vi "process_DAQ.vi"(8 "error in (no error)":errorcluster) -> (0 "error out":errorcluster)   [LabVIEW 2010]
uses:
  typedefs/control_daq_enum.ctl
  typedefs/data_array.ctl
  typedefs/acquisition_parameters_cluster.ctl
  typedefs/stimulation_parameters.ctl
  C:/Program Files (x86)/National Instruments/LabVIEW 2010/vi.lib/ULx/ULx_LV.dll
  Program Files (x86)/National Instruments/LabVIEW 2010/vi.lib/ULx/ULx_LV.dll
  <vilib>/ULx/Read.llb/ULx Read (Analog 2D DBL NChan NSamp).vi
panel:
  out "Package start time":timestamp format="%<%.3X>T"
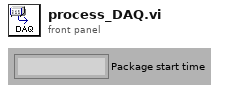
[diagram p1: front panel]
types:
  T1 = typedef "control_daq_enum.ctl" = enum16{"Init", "GetCont", "GetNoSamples", "Stop", "Quit"}
  T2 = cluster{"Control DAQ Enum":T1, "variant":variant}
  T3 = typedef "data_array.ctl" = waveform(dbl)[]
  T4 = typedef "acquisition_parameters_cluster.ctl" = cluster{"Physical channels":refnum<k21>, "Shutter line":refnum<k21>, "Clock source":i32, "Triggered?":bool, "Sample rate":dbl, "Pixels to integrate":i32, "Effective data rate":dbl, "Read chunk size":i32, "Samples to read":i32, "Run mode":enum32{"Continuously", "Fixed sample number"}}
  T5 = typedef "stimulation_parameters.ctl" = cluster{"Physical channel":tag, "Write chunk size":i32, "Sample rate":dbl, "Stim onset":dbl, "Stim frequency":dbl, "ON time":dbl, "OFF time":dbl, "Repetitions":dbl}
  T6 = cluster{"Acquisition parameters":T4, "Stimulation parameters":T5}
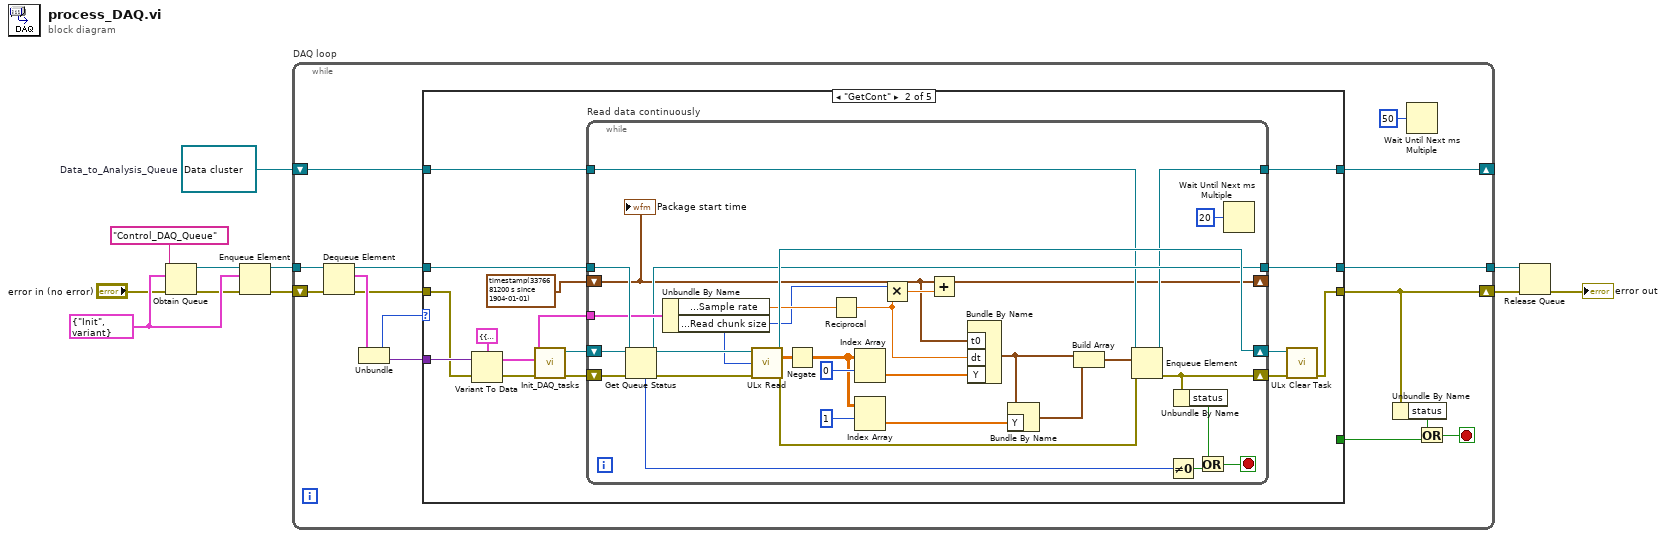
[diagram p0: block diagram]
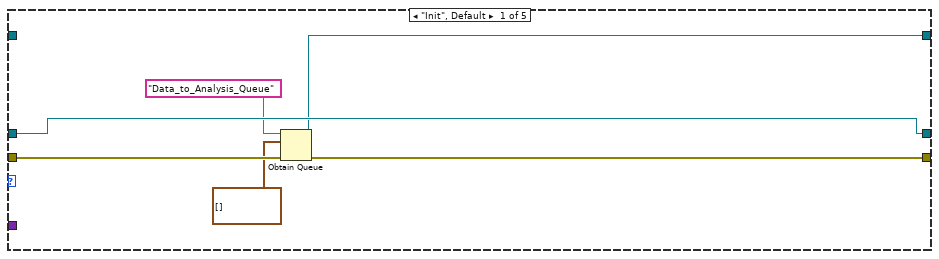
[diagram p2: hidden frame]
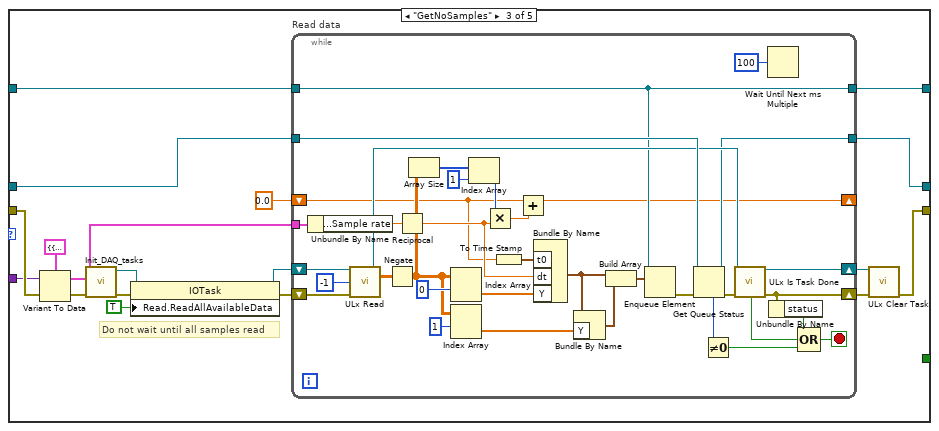
[diagram p3: hidden frame]
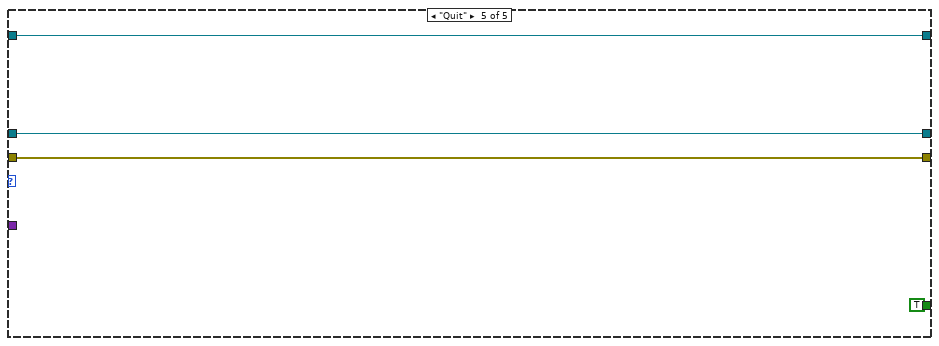
[diagram p5: hidden frame]
diagram:
  w1 = refnum<queue> refnum  # Data_to_Analysis_Queue
  w11 = T2 {"Control DAQ Enum"=enum."Init", "variant"=variant} ("ControlDAQ state cluster")
  n1 = Obtain Queue(name (unnamed)="Control_DAQ_Queue", element data type=w11, error in (no error)="error in (no error)") -> (queue out=w7:refnum<queue>, error out=w9:errorcluster)  [unwired: 2 in, 1 out]
  n2 = Enqueue Element(queue=w7, element=w11, error in (no error)=w9) -> (queue out=w8:refnum<queue>, error out=w10:errorcluster)  [unwired: 1 in, 1 out]
  n3 = while "DAQ loop" {
    shift-right: [w19] -> w6
    shift-left: w10 -> [w25]
    tunnel: w8 -> [w26]
    tunnel: [w15] -> w5
    shift-right: [w13] -> _
    shift-left: w1 -> [w14]
    stop <- w17 stop-if-true
    n4 = Dequeue Element(queue=w26, error in (no error)=w25) -> (queue out=w24:refnum<queue>, element=w23:T2, error out=w21:errorcluster)  [unwired: 1 in, 1 out]
    n5 = Unbundle(w23) -> ("Control DAQ Enum"=w16:T1, "variant"=w22:variant)
    n6 = case shown="\"GetCont\"" w16 {
      tunnel: w24 -> [w32 w47 w91 w134 w137]
      tunnel: w22 -> [_ w46 w92 _ _]
      tunnel: w21 -> [w31 w45 w93 w135 w138]
      tunnel: [w29 w34 w90 w135 w138] -> w19
      tunnel: [_ _ _ _ TRUE] -> w20
      tunnel: [w32 w38 w82 w134 w137] -> w15
      tunnel: w14 -> [_ w37 w81 w133 w136]
      tunnel: [w27 w36 w80 w133 w136] -> w13
      frame "Init", Default {
        n7 = Obtain Queue(name (unnamed)="Data_to_Analysis_Queue", element data type=T3 [] ("Data cluster"), error in (no error)=w31) -> (queue out=w27:refnum<queue>, error out=w29:errorcluster)  [unwired: 2 in, 1 out]
      }
      frame "GetCont" {
        n8 = Variant To Data(error in=w45, Variant=w46, type=T6 {"Acquisition parameters"={"Physical channels"="", "Shutter line"="", "Clock source"=0, "Triggered?"=FALSE, "Sample rate"=0.0, "Pixels to integrate"=0, "Effective data rate"=0.0, "Read chunk size"=0, "Samples to read"=0, "Run mode"=enum."Continuously"}, "Stimulation parameters"={"Physical channel"="", "Write chunk size"=0, "Sample rate"=0.0, "Stim onset"=0.0, "Stim frequency"=0.0, "ON time"=0.0, "OFF time"=0.0, "Repetitions"=0.0}} ("output cluster")) -> (error out=w44:errorcluster, data=w41:T6)
        n9 = call "Init_DAQ_tasks.vi"("error in"=w44, "Parameter cluster"=w41) -> ("error out"=w43:errorcluster, "Acq task out"=w42:refnum<k24>)  [unwired: 6 in]
        n10 = while "Read data continuously" {
          shift-right: [w65] -> w39
          shift-left: w43 -> [w69]
          tunnel: w41 -> [w72]
          shift-right: [w73] -> w40
          shift-left: w42 -> [w76]
          shift-right: [w51] -> _
          shift-left: timestamp(3376681200 s since 1904-01-01) ("time stamp") -> [w48]
          tunnel: w37 -> [w70]
          tunnel: [w67] -> w36
          tunnel: w47 -> [w78]
          tunnel: [w71] -> w38
          stop <- w74 stop-if-true
          n11 = Get Queue Status(queue=w78, error in (no error)=w69) -> (queue out=w71:refnum<queue>, error out=w66:errorcluster, # elements in queue=w77:i32)  [unwired: 1 in, 5 out]
          n12 = Unbundle By Name(w72) -> ("Acquisition parameters.Sample rate"=w57:dbl, "Acquisition parameters.Read chunk size"=w49:i32)
          n13 = call-poly <vilib>:"ULx Read.vi"("task in"=w76, "number of samples per channel"=w49, "error in"=w66) -> ("task out"=w73:refnum<k24>, "data"=w68:dbl[][], "error out"=w54:errorcluster)  [unwired: 10 in]
          n14 = Negate(x=w68) -> (-x=w60:dbl[][])
          n15 = Reciprocal(x=w57) -> (1/x=w50:dbl)
          n16 = Index Array(array=w60, index (row)=0) -> (element=w56:dbl[])  [unwired: 1 in]
          n17 = Index Array(array=w60, index (row)=1) -> (element=w59:dbl[])  [unwired: 1 in]
          n18 = Multiply(x=w49, y=w50) -> (x*y=w53:dbl)
          n19 = Add(x=w48, y=w53) -> (x+y=w51:timestamp)
          n20 = Bundle By Name("t0"=w48, "dt"=w50, "Y"=w56) -> (w55:waveform(dbl))  [unwired: 1 in]
          n21 = Bundle By Name(cluster=w55, "Y"=w59) -> (w58:waveform(dbl))
          n22 = Build Array(w55, w58) -> (w52:waveform(dbl)[])
          n23 = Enqueue Element(queue=w70, element=w52, error in (no error)=w54) -> (queue out=w67:refnum<queue>, error out=w65:errorcluster)  [unwired: 1 in, 1 out]
          n24 = Not Equal To 0?(x=w77) -> (x != 0?=w75:bool)
          n25 = Unbundle By Name(w65) -> ("status"=w64:bool)
          n26 = Or(x=w64, y=w75) -> (x .or. y?=w74:bool)
          n27 = Wait Until Next ms Multiple(millisecond multiple=u32 20) -> ()  [unwired: 1 out]
          "Package start time" <- w48
        }
        n28 = call <vilib>:"ULx Clear Task.vi"("task in"=w40, "error in"=w39) -> ("error out"=w34:errorcluster)  [unwired: 13 in]
      }
      frame "GetNoSamples" {
        # "Do not wait until all samples read"
        n29 = Variant To Data(error in=w93, Variant=w92, type=T6 {"Acquisition parameters"={"Physical channels"="", "Shutter line"="", "Clock source"=0, "Triggered?"=FALSE, "Sample rate"=0.0, "Pixels to integrate"=0, "Effective data rate"=0.0, "Read chunk size"=0, "Samples to read"=0, "Run mode"=enum."Continuously"}, "Stimulation parameters"={"Physical channel"="", "Write chunk size"=0, "Sample rate"=0.0, "Stim onset"=0.0, "Stim frequency"=0.0, "ON time"=0.0, "OFF time"=0.0, "Repetitions"=0.0}} ("output cluster")) -> (error out=w96:errorcluster, data=w84:T6)
        n30 = call "Init_DAQ_tasks.vi"("error in"=w96, "Parameter cluster"=w84) -> ("error out"=w87:errorcluster, "Acq task out"=w89:refnum<k24>)  [unwired: 6 in]
        n31 = property class="IOTask"(reference=w89, error in=w87, "Read.ReadAllAvailableData"=TRUE) -> (reference out=w88:refnum<k24>, error out=w86:errorcluster)
        n32 = while "Read data" {
          shift-right: [w124] -> w94
          shift-left: w86 -> [w130]
          shift-right: [w126] -> w95
          shift-left: w88 -> [w129]
          tunnel: w84 -> [w119]
          shift-right: [w98] -> _
          shift-left: 0.0 -> [w97]
          tunnel: w91 -> [w132]
          tunnel: [w118] -> w82
          tunnel: w81 -> [w117]
          tunnel: [w117] -> w80
          stop <- w120 stop-if-true
          n33 = Unbundle By Name(w119) -> ("Acquisition parameters.Sample rate"=w112:dbl)
          n34 = call-poly <vilib>:"ULx Read.vi"("task in"=w129, "number of samples per channel"=-1, "error in"=w130) -> ("task out"=w127:refnum<k24>, "data"=w115:dbl[][])  [unwired: 10 in, 1 out]
          n35 = Negate(x=w115) -> (-x=w105:dbl[][])
          n36 = Reciprocal(x=w112) -> (1/x=w101:dbl)
          n37 = Array Size(array=w105) -> (size(s)=w104:i32[])
          n38 = Index Array(array=w105, index (row)=0) -> (element=w111:dbl[])  [unwired: 1 in]
          n39 = Index Array(array=w105, index (row)=1) -> (element=w110:dbl[])  [unwired: 1 in]
          n40 = Index Array(array=w104, index=1) -> (element=w102:i32)
          n41 = Multiply(x=w102, y=w101) -> (x*y=w100:dbl)
          n42 = To Time Stamp(1:w97) -> (0:w99:timestamp)
          n43 = Add(x=w97, y=w100) -> (x+y=w98:dbl)
          n44 = Bundle By Name("t0"=w99, "dt"=w101, "Y"=w111) -> (w109:waveform(dbl))  [unwired: 1 in]
          n45 = Bundle By Name(cluster=w109, "Y"=w110) -> (w108:waveform(dbl))
          n46 = Build Array(w109, w108) -> (w106:waveform(dbl)[])
          n47 = Enqueue Element(queue=w117, element=w106) -> (error out=w116:errorcluster)  [unwired: 2 in, 2 out]
          n48 = Get Queue Status(queue=w132, error in (no error)=w116) -> (queue out=w118:refnum<queue>, error out=w125:errorcluster, # elements in queue=w131:i32)  [unwired: 1 in, 5 out]
          n49 = Not Equal To 0?(x=w131) -> (x != 0?=w123:bool)
          n50 = call <vilib>:"ULx Is Task Done.vi"("task in"=w127, "error in"=w125) -> ("task out"=w126:refnum<k24>, "task done?"=w122:bool, "error out"=w124:errorcluster)  [unwired: 11 in]
          n51 = Wait Until Next ms Multiple(millisecond multiple=u32 100) -> ()  [unwired: 1 out]
          n52 = Unbundle By Name(w124) -> ("status"=w121:bool)
          n53 = Compound Arithmetic op=OR(w121, w122, w123) -> (w120:bool)
        }
        n54 = call <vilib>:"ULx Clear Task.vi"("task in"=w95, "error in"=w94) -> ("error out"=w90:errorcluster)  [unwired: 13 in]
      }
      frame "Stop" {
      }
      frame "Quit" {
      }
    }
    n55 = Unbundle By Name(w19) -> ("status"=w18:bool)
    n56 = Wait Until Next ms Multiple(millisecond multiple=u32 50) -> ()  [unwired: 1 out]
    n57 = Or(x=w18, y=w20) -> (x .or. y?=w17:bool)
  }
  n58 = Release Queue(queue=w5, error in (no error)=w6) -> (error out=→"error out":errorcluster)  [unwired: 1 in, 2 out]
